vi "Wait.vi"(7 "milliseconds to wait":u32=250, 11 "Error In":errorcluster) -> (3 "Error Out":errorcluster)   [LabVIEW 2024]
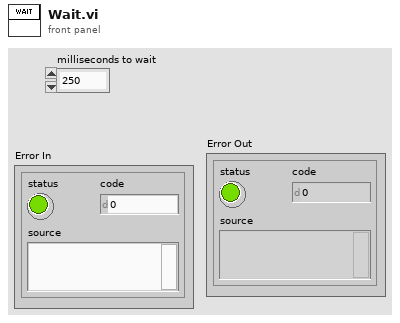
[diagram p1: front panel]
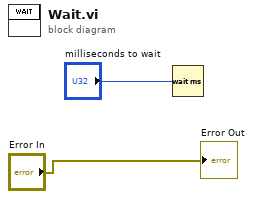
[diagram p0: block diagram]
diagram:
  n1 = Wait (ms)(milliseconds to wait="milliseconds to wait") -> ()  [unwired: 1 out]
  "Error Out" <- "Error In"
